vi "IHL_HS Stream Sample Data Notifier.vi"(8 "error in (no error)":errorcluster, 10 "Create New?":bool) -> (0 "error out":errorcluster, 2 "Sample Data notifier out":refnum<notifier>)   [LabVIEW 2015, in "Tool Module.lvlib"]
uses:
  Tool Module.lvlib
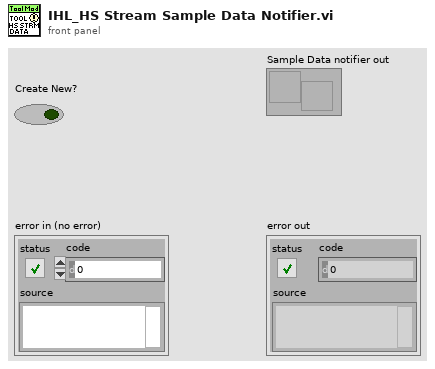
[diagram p1: front panel]
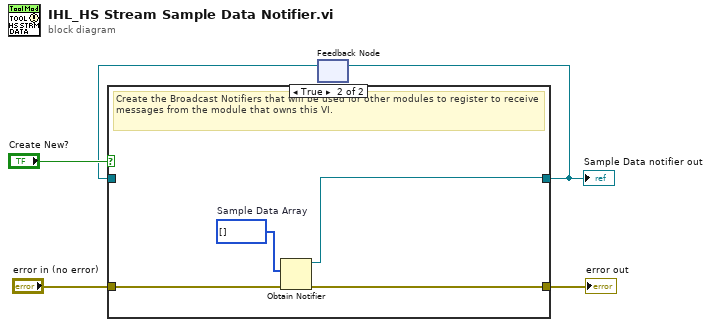
[diagram p0: block diagram]
diagram:
  n1 = feedback #1() -> (w1:refnum<notifier>)  [unwired: 1 in]
  n2 = case shown="True" "Create New?" {
    tunnel: [w7 w8] -> w2
    tunnel: [w6 w10] -> w5
    tunnel: "error in (no error)" -> [w6 w9]
    tunnel: w1 -> [w7 _]
    frame False {
      # "Obtain the Broadcast notifiers that were created in a previous call to this VI."
    }
    frame True {
      w11 = u32[] []  # Sample Data Array
      # "Create the Broadcast Notifiers that will be used for other modules to register to receive messages from the module that owns this VI."
      n3 = Obtain Notifier(notification data type=w11, error in (no error)=w9) -> (notifier out=w8:refnum<notifier>, error out=w10:errorcluster)  [unwired: 2 in, 1 out]
    }
  }
  "error out" <- w5
  "Sample Data notifier out" <- w2
  n4 = feedback-in #1(w2) -> ()
